vi "update LEDs.vi"(8 "error in (no error)":errorcluster, 11 "Cobolt in":refnum<class "Cobolt.lvclass">) -> (0 "error out":errorcluster, 3 "Cobolt out":refnum<class "Cobolt.lvclass">)   [LabVIEW 2012, in "Cobolt.lvclass"]
uses:
  Cobolt.lvclass
  Cobolt.lvclass/Cobolt.ctl
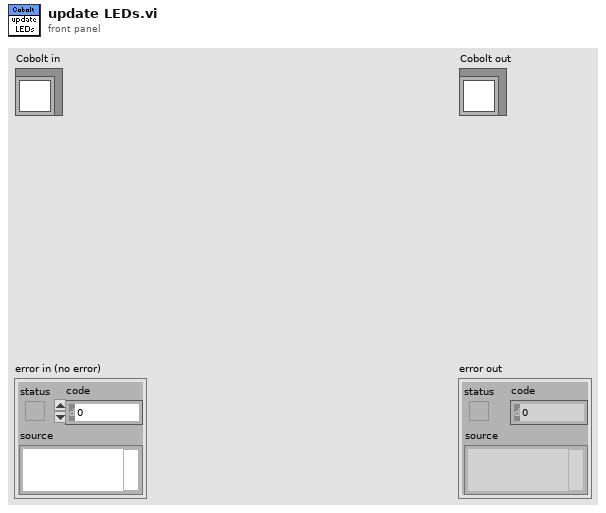
[diagram p1: front panel]
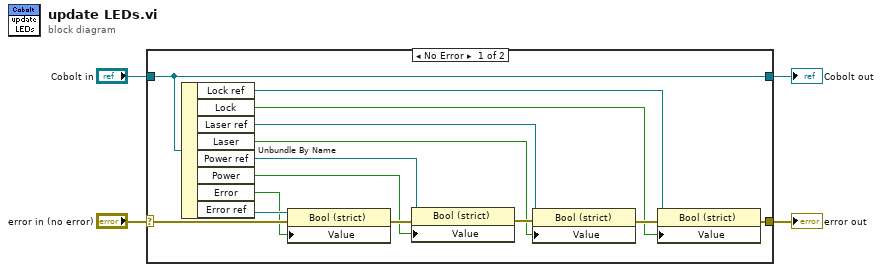
[diagram p0: block diagram]
diagram:
  n1 = case shown="No Error" "error in (no error)" {
    selector: "error in (no error)" -> [w17 w20]
    tunnel: [w8 w20] -> w3
    tunnel: [w18 w19] -> w1
    tunnel: "Cobolt in" -> [w18 w19]
    frame No Error {
      n2 = Unbundle By Name(w18) -> ("Lock ref"=w6:refnum<vi>, "Lock"=w5:bool, "Laser ref"=w10:refnum<vi>, "Laser"=w9:bool, "Power ref"=w11:refnum<vi>, "Power"=w12:bool, "Error"=w15:bool, "Error ref"=w16:refnum<vi>)
      n3 = property class="Bool (strict)"(reference=w16, error in=w17, "Value"=w15) -> (error out=w14:errorcluster)  [unwired: 1 out]
      n4 = property class="Bool (strict)"(reference=w11, error in=w14, "Value"=w12) -> (error out=w13:errorcluster)  [unwired: 1 out]
      n5 = property class="Bool (strict)"(reference=w10, error in=w13, "Value"=w9) -> (error out=w7:errorcluster)  [unwired: 1 out]
      n6 = property class="Bool (strict)"(reference=w6, error in=w7, "Value"=w5) -> (error out=w8:errorcluster)  [unwired: 1 out]
    }
    frame Error {
    }
  }
  "error out" <- w3
  "Cobolt out" <- w1
